vi "P9374A NA scpi.vi"() -> ()   [LabVIEW 2021]
uses:
  <instrlib>/Agilent NA/Agilent NA.lvlib
panel:
  out "Val":string="Keysight Technologies,P9374A,MY57212430,A.13.10.05\n"
  in  "Command":string="*IDN?"
  out "error out":errorcluster {"code" format="%.0x"}
  in  "resource name":refnum<k15>="P9374A" caption="resource string"
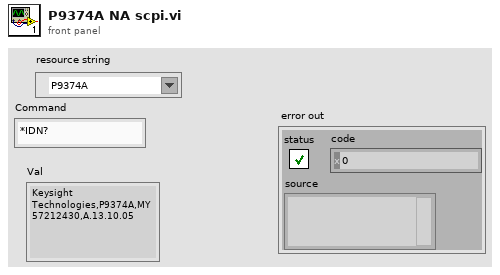
[diagram p1: front panel]
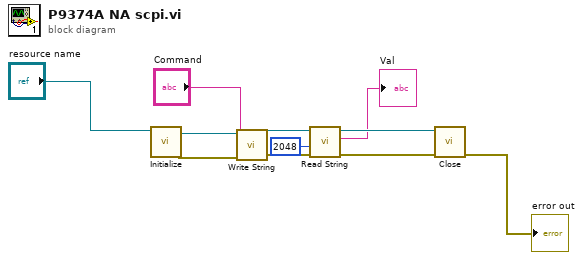
[diagram p0: block diagram]
diagram:
  n1 = call <instrlib>:"Initialize.vi"("resource name"="resource name") -> ("error out"=w9:errorcluster, "instrument handle out"=w8:refnum<k15>)  [unwired: 9 in]
  n2 = call <instrlib>:"Write String.vi"("error in (no error)"=w9, "Command"="Command", "instrument handle"=w8) -> ("error out"=w5:errorcluster, "instrument handle out"=w6:refnum<k15>)  [unwired: 7 in]
  n3 = call <instrlib>:"Read String.vi"("error in (no error)"=w5, "ValBufferSize"=2048, "instrument handle"=w6) -> ("error out"=w4:errorcluster, "Val"=→"Val":string, "instrument handle out"=w3:refnum<k15>)  [unwired: 6 in]
  n4 = call <instrlib>:"Close.vi"("error in (no error)"=w4, "instrument handle"=w3) -> ("error out"=→"error out":errorcluster)  [unwired: 9 in]
